vi "Create BIN list by Bin Count.vi"(9 "Number of Bins":dbl, 10 "Min":dbl, 11 "Max":dbl) -> (3 "Bins":T1(array[cluster]) {"upper" format="%0.2f"; "lower" format="%0.2f"})   [LabVIEW 2011]
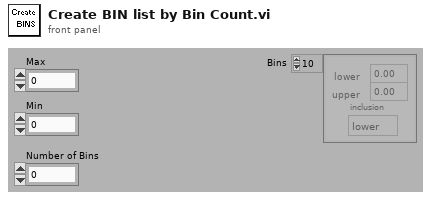
[diagram p1: front panel]
types:
  T1 = cluster{"lower":dbl, "upper":dbl, "inclusion":enum32{"lower", "upper", "both", "neither"}}[]
  T2 = cluster{"lower":dbl, "upper":dbl, "inclusion":enum32{"lower", "upper", "both", "neither"}}
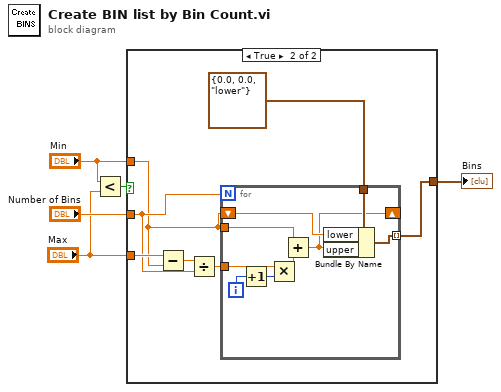
[diagram p0: block diagram]
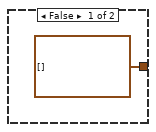
[diagram p2: hidden frame]
diagram:
  n1 = Less?(x="Min", y="Max") -> (x < y?=w1:bool)
  n2 = case shown="True" w1 {
    tunnel: [T1 [] w12] -> w5
    tunnel: "Number of Bins" -> [_ w9]
    tunnel: "Min" -> [_ w7]
    tunnel: "Max" -> [_ w11]
    frame False {
    }
    frame True {
      n3 = Subtract(x=w11, y=w7) -> (x-y=w10:dbl)
      n4 = Divide(x=w10, y=w9) -> (x/y=w8:dbl)
      n5 = for {
        N: w9 -> [_]
        tunnel: T2 {"lower"=0.0, "upper"=0.0, "inclusion"=enum."lower"} -> [w22]
        tunnel: [w21] -> w12 mode=indexing
        tunnel: w7 -> [w18]
        tunnel: w8 -> [w20]
        shift-right: [w15] -> _
        shift-left: w7 -> [w16]
        i -> [w19]
        n6 = Increment(x=w19) -> (x+1=w14:i32)
        n7 = Multiply(x=w20, y=w14) -> (x*y=w17:dbl)
        n8 = Add(x=w18, y=w17) -> (x+y=w15:dbl)
        n9 = Bundle By Name(cluster=w22, "lower"=w16, "upper"=w15) -> (w21:T2)
      }
    }
  }
  "Bins" <- w5
